vi "CPP_AeroprobePerBlock.vi"() -> (5 "Plug in titles":string[](array[string]), 7 "Plug in values":string[](array[string]))   [LabVIEW 2010]
uses:
  Applications/EnFloSW/EnFloCPPHybrid/Anemometry/Anemometry Sub Vis/Globals/Meas_global.vi
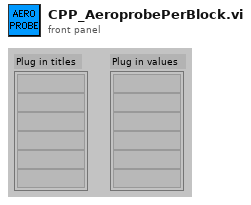
[diagram p1: front panel]
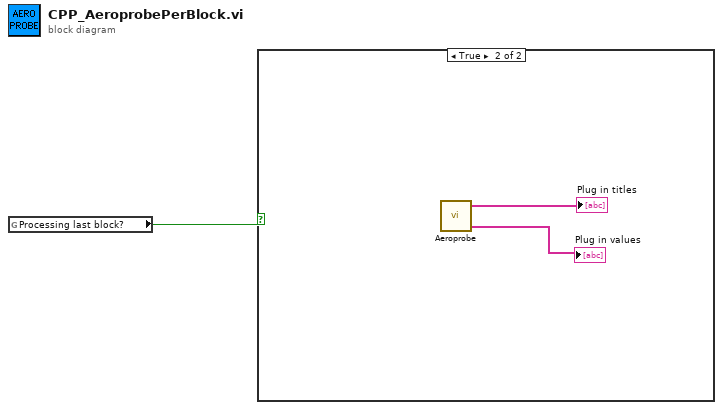
[diagram p0: block diagram]
diagram:
  n1 = global read "Meas_global.vi" "Processing last block?"() -> (w1:bool)
  n2 = case shown="True" w1 {
    frame False {
    }
    frame True {
      n3 = call "Aeroprobe.vi"() -> ("Plug in titles"=→"Plug in titles":string[], "Plug in values"=→"Plug in values":string[])  [unwired: 6 in]
    }
  }
